vi "Untitled 1.vi"() -> ()   [LabVIEW 2020, in "Detector Class.lvclass"]
uses:
  Detector Class.lvclass
  PRIME Detector/PRIME Detector.lvclass
  C:/Development/prime/Prime-RIMAS/Detector/Detector Class/Detector Class.lvclass
  C:/Development/prime/Prime-RIMAS/Detector/Detector Class/PRIME Detector/PRIME Detector.lvclass
  Detector Image typedef cluster.ctl
panel:
  out "Images":T1[](array[typedef]) {"Detector #" items=["None", "YJ", "HK"]}
  out "Message Log":string
  out "PRIME Detector out":refnum<class "PRIME Detector.lvclass">
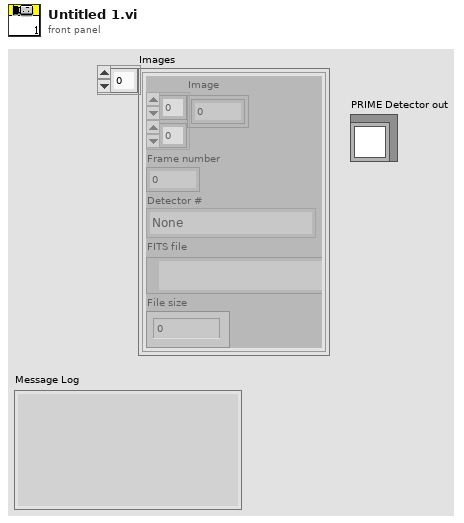
[diagram p1: front panel]
types:
  T1 = typedef "Detector Class.lvclass/Detector Image typedef cluster.ctl" = cluster{"Image":sgl[][], "Frame number":i32, "Detector #":u16, "FITS file":path, "File size":i64}
  T2 = typedef "RIMAS Observation Config.ctl" = cluster{"Exp Time Short":dbl, "# of Frames":dbl, "Exp Time Long":dbl, "# of Groups":dbl, "Object Name":string, "Object":string, "Obs Type":string, "Image Type":string, "Observer":string, "Observer Affiliation":string}
  T3 = typedef "PRIME Detector cluster Status.ctl" = cluster{"Cmd Start Time":timestamp, "Command":string, "Complete?":bool, "Cmd Complete Time":timestamp, "Exp Time Remaining":dbl, "Total Frames":i32, "Exp Frames":cluster{"CAMERA0":string[], "CAMERA1":string[], "CAMERA2":string[], "CAMERA3":string[]}, "Intermediate Frames":cluster{"CAMERA0":string[], "CAMERA1":string[], "CAMERA2":string[], "CAMERA3":string[]}, "Final Reduced Frame":cluster{"CAMERA0":string, "CAMERA1":string, "CAMERA2":string, "CAMERA3":string}}
  T4 = cluster{"CAMERA0":string[], "CAMERA1":string[], "CAMERA2":string[], "CAMERA3":string[]}
  T5 = cluster{"CAMERA0":string, "CAMERA1":string, "CAMERA2":string, "CAMERA3":string}
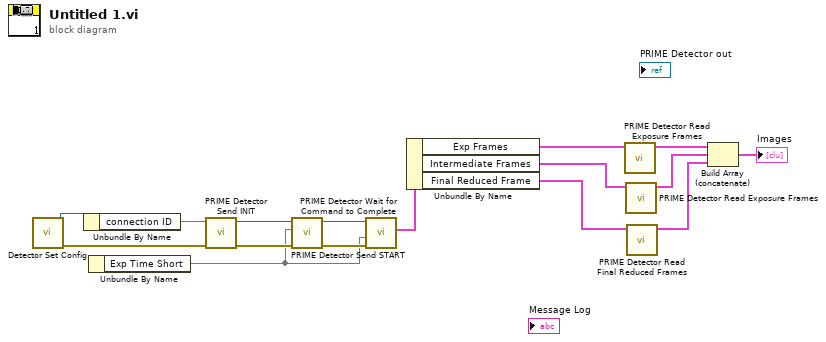
[diagram p0: block diagram]
diagram:
  n1 = call-dynamic "Detector Set Config.vi"() -> ("error out"=w17:errorcluster, "PRIME Detector out"=w18:refnum<class "PRIME Detector.lvclass">, "error in (no error)"=w19:errorcluster, "PRIME Detector in"=w16:refnum<class "PRIME Detector.lvclass">)  [unwired: 8 in]
  n2 = Unbundle By Name(w18) -> ("connection ID"=w20)
  n3 = Unbundle By Name() -> (w12:T2, "Exp Time Short"=w10)
  n4 = call "PRIME Detector Send INIT.vi"("error in (no error)"=w17, "connection ID"=w20) -> ("error out"=w13:errorcluster, "connection ID out"=w14:refnum<k5>)  [unwired: 8 in]
  n5 = call "PRIME Detector Send START.vi"("error in (no error)"=w13, "Exposure Time"=w10, "connection ID"=w14) -> ("error out"=w11:errorcluster, "connection ID out"=w9:refnum<k5>)  [unwired: 7 in]
  n6 = call "PRIME Detector Wait for Command to Complete.vi"("error in (no error)"=w11, "Exp Time"=w10, "connection ID"=w9) -> ("Status"=w8:T3)  [unwired: 6 in, 2 out]
  n7 = Unbundle By Name(w8) -> ("Exp Frames"=w7:T4, "Intermediate Frames"=w6:T4, "Final Reduced Frame"=w5:T5)
  n8 = call "PRIME Detector Read Exposure Frames.vi"("Exp Frames"=w7) -> ("Images"=w4:T1[])  [unwired: 10 in]
  n9 = call "PRIME Detector Read Exposure Frames.vi"("Exp Frames"=w6) -> ("Images"=w3:T1[])  [unwired: 10 in]
  n10 = call "PRIME Detector Read Final Reduced Frames.vi"("Final Reduced Frame"=w5) -> ("Images"=w2:T1[])  [unwired: 10 in]
  n11 = Build Array (concatenate)(w4, w3, w2) -> (→"Images":T1[])
